vi "TcA07-006_CastFromLabVIEWObject.vi"(1 "Input buffer":T3="1", 3 "Invocation info":T2, 5 "error in (no error)":errorcluster, 6 "Add log to result?":bool) -> (16 "Test Data":T1 {"Numeric Measurement" format="%.2f"}, 19 "error out":errorcluster)   [LabVIEW 2020]
doc: "Test case template."
uses:
  Shared/Support_InputBuffer.ctl
  Shared/Support_InvocationInfo.ctl
  Shared/Support_TestData.ctl
  <vilib>/addons/_AddQ/G#Object/G#Object.lvclass
  TestClasses/G#SubClass1_class/G#SubClass1.lvclass
panel:
  in  "Test name":string="TcA07-006 Cast from LV object"
  out "Test result":bool
  out "Result":string
  # "Reference casting from a LabVIEW object works."
  # "Sub test case"
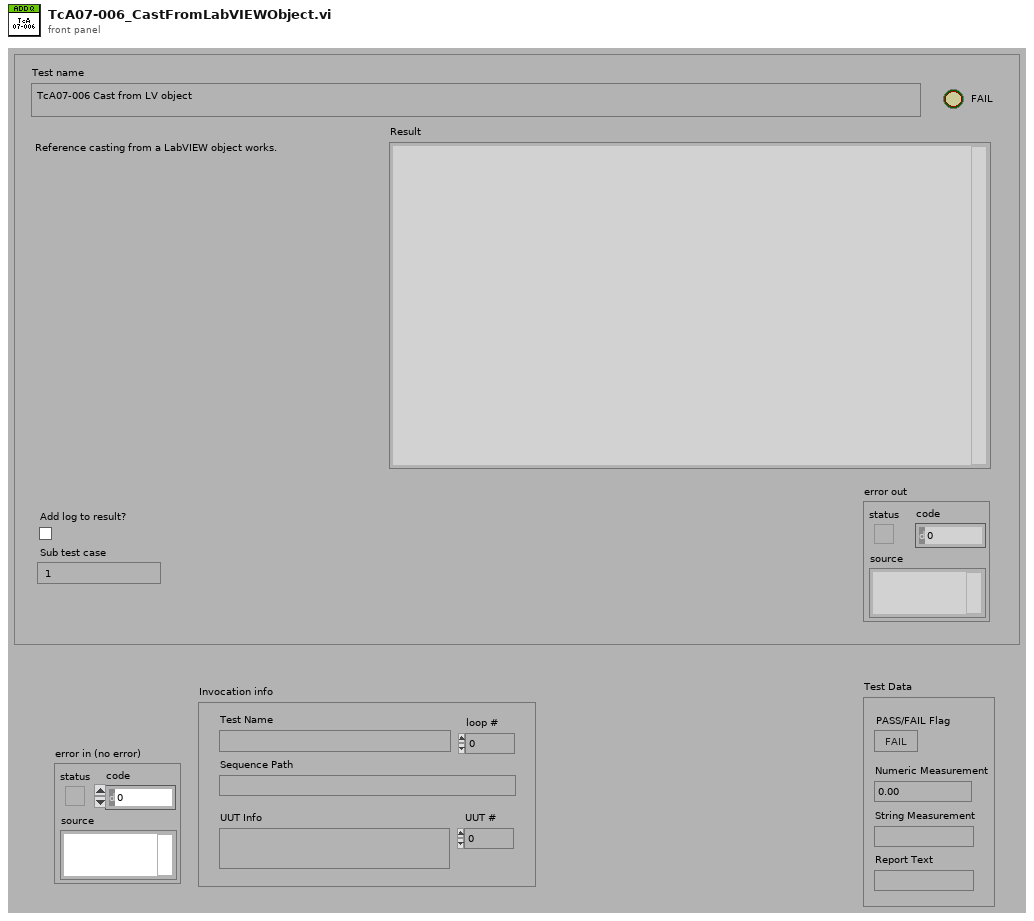
[diagram p1: front panel]
types:
  T1 = typedef "Support_TestData.ctl" = cluster{"PASS/FAIL Flag":bool, "Numeric Measurement":dbl, "String Measurement":string, "Report Text":string}
  T2 = typedef "Support_InvocationInfo.ctl" = cluster{"UUT #":i32, "loop #":i32, "UUT Info":string, "Test Name":string, "Sequence Path":path}
  T3 = typedef "Support_InputBuffer.ctl" = string
  T4 = typedef "Support_ResultType.ctl" = cluster{"Pass":bool, "Comment":string, "MeasurementValue":dbl}
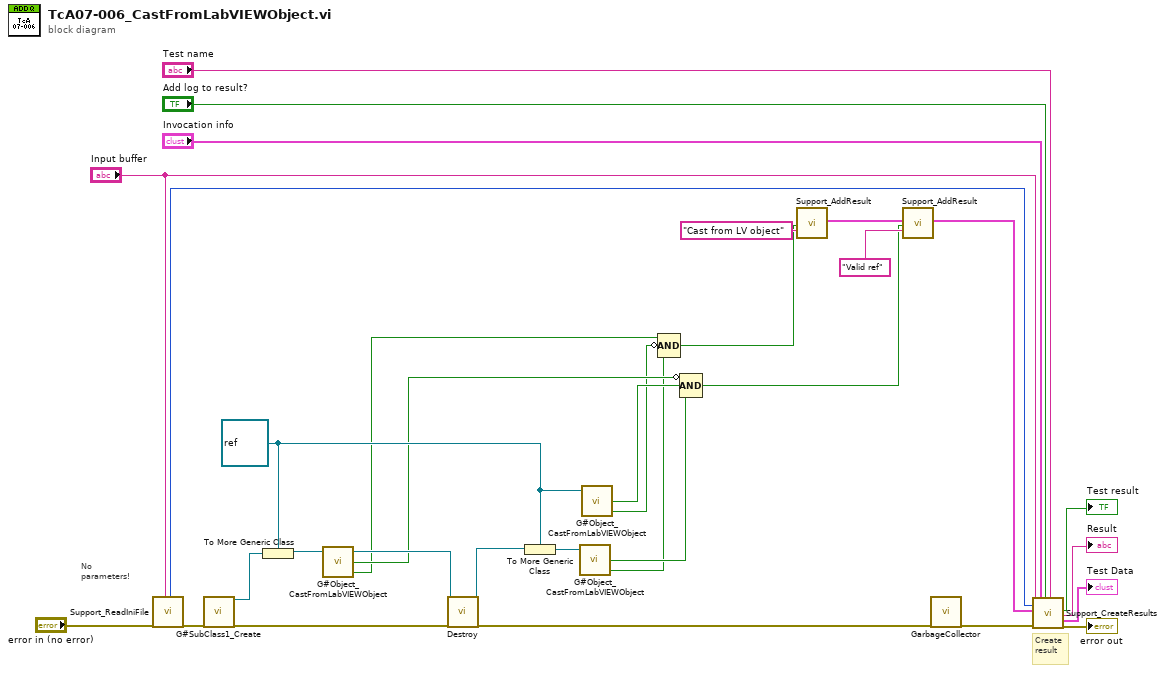
[diagram p0: block diagram]
diagram:
  w9 = refnum<class> refnum ("LabVIEWObject in")
  # "No\nparameters!"
  # "Create\nresult"
  n1 = call "Support_ReadIniFile.vi"("error in (no error)"="error in (no error)", "Sub test case"="Input buffer") -> ("Timer start"=w23:u32, "error out"=w21:errorcluster)  [unwired: 10 in, 6 out]
  n2 = call "G#SubClass1_Create.vi"("error in (no error)"=w21) -> ("reference out"=w20:refnum<class "G#SubClass1.lvclass">, "error out"=w18:errorcluster)  [unwired: 16 in, 1 out]
  n3 = To More Generic Class(target class=w9, reference=w20) -> (generic class reference=w19:refnum<class>)
  n4 = call <vilib>:"G#Object_CastFromLabVIEWObject.vi"("LabVIEWObject in"=w19) -> ("is of G#Object?"=w4:bool, "not a refnum?"=w8:bool, "reference out"=w17:refnum<class "G#Object.lvclass">)  [unwired: 2 in]
  n5 = call-dynamic "Destroy.vi"("reference in"=w17, "error in (no error)"=w18) -> ("reference out"=w16:refnum<class "G#Object.lvclass">, "error out"=w14:errorcluster)  [unwired: 16 in]
  n6 = To More Generic Class(target class=w9, reference=w16) -> (generic class reference=w15:refnum<class>)
  n7 = call <vilib>:"G#Object_CastFromLabVIEWObject.vi"("LabVIEWObject in"=w15) -> ("is of G#Object?"=w2:bool, "not a refnum?"=w6:bool)  [unwired: 2 in, 1 out]
  n8 = call <vilib>:"G#Object_CastFromLabVIEWObject.vi"("LabVIEWObject in"=w9) -> ("is of G#Object?"=w3:bool, "not a refnum?"=w7:bool)  [unwired: 2 in, 1 out]
  n9 = Compound Arithmetic op=AND(w4, invert w3, w2) -> (w1:bool)
  n10 = Compound Arithmetic op=AND(invert w8, w7, w6) -> (w5:bool)
  n11 = call "Support_AddResult.vi"("Pass"=w1, "Comment"="Cast from LV object") -> ("Results out"=w11:T4[])  [unwired: 17 in]
  n12 = call "Support_AddResult.vi"("Results in"=w11, "Pass"=w5, "Comment"="Valid ref") -> ("Results out"=w12:T4[])  [unwired: 16 in]
  n13 = call <vilib>:"GarbageCollector.vi"("error in (no error)"=w14) -> ("error out"=w22:errorcluster)  [unwired: 16 in, 2 out]
  n14 = call "Support_CreateResults.vi"("Sub test case"="Input buffer", "Timer start"=w23, "Results"=w12, "error in (no error)"=w22, "Invocation info"="Invocation info", "Add log to result?"="Add log to result?", "Test name"="Test name") -> ("Pass/fail flag"=→"Test result":bool, "Result"=→"Result":string, "Test Data"=→"Test Data":T1, "error out"=→"error out":errorcluster)  [unwired: 9 in]
